vi "FT10_Date and Time String.vi"(11 "to UTC":bool) -> (3 "Date & Time string":string)   [LabVIEW 2015]
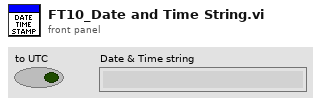
[diagram p1: front panel]
types:
  T1 = typedef "LVDateTimeRec.ctl" = cluster{"fractional second":dbl, "second":i32, "minute":i32, "hour":i32, "day of month":i32, "month":i32, "year":i32, "day of week":i32, "day of year":i32, "DST":i32}
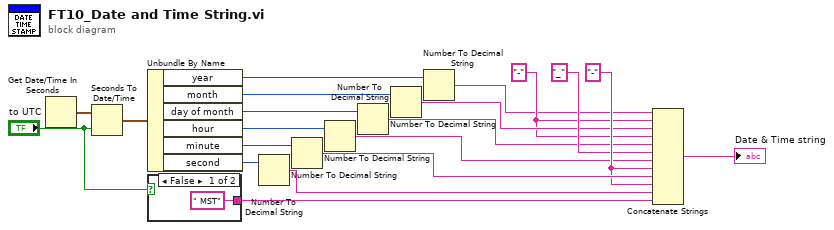
[diagram p0: block diagram]
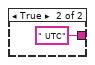
[diagram p2: hidden frame]
diagram:
  w16 = "-" ("string")
  w11 = "-" ("string")
  n1 = Get Date/Time In Seconds() -> (seconds since 1Jan1904=w1:timestamp)
  n2 = Seconds To Date/Time(time stamp (now)=w1, to UTC (F)="to UTC") -> (date time rec=w2:T1)
  n3 = Unbundle By Name(w2) -> ("year"=w3:i32, "month"=w4:i32, "day of month"=w5:i32, "hour"=w6:i32, "minute"=w7:i32, "second"=w8:i32)
  n4 = case shown="False" "to UTC" {
    tunnel: [" MST" ("string") " UTC" ("string")] -> w20
    frame False {
    }
    frame True {
    }
  }
  n5 = Number To Decimal String(number=w8) -> (decimal integer string=w18:string)  [unwired: 1 in]
  n6 = Number To Decimal String(number=w7) -> (decimal integer string=w17:string)  [unwired: 1 in]
  n7 = Number To Decimal String(number=w6) -> (decimal integer string=w15:string)  [unwired: 1 in]
  n8 = Number To Decimal String(number=w5) -> (decimal integer string=w13:string)  [unwired: 1 in]
  n9 = Number To Decimal String(number=w4) -> (decimal integer string=w12:string)  [unwired: 1 in]
  n10 = Number To Decimal String(number=w3) -> (decimal integer string=w10:string)  [unwired: 1 in]
  n11 = Concatenate Strings(w10, w11, w12, w11, w13, "_" ("string"), w15, w16, w17, w16, w18, w20) -> (→"Date & Time string":string)
